vi "PlatMods Artificial.vi"(8 "error in (no error)":errorcluster) -> (0 "error out":errorcluster, 3 "PlatMods":T1)   [LabVIEW 2021, in "RocketPlot.lvlib"]
uses:
  RocketPlot.lvlib
  TypeDefs/PlatMods.ctl
  <vilib>/Utility/inputDevices.llb/keyboardAcquire.vi
  <vilib>/Utility/inputDevices.llb/closeKeyboard.vi
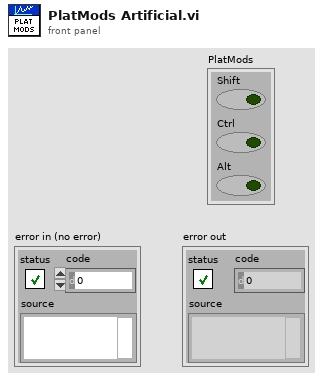
[diagram p1: front panel]
types:
  T1 = typedef "RocketPlot.lvlib/PlatMods.ctl" = cluster{"Shift":bool, "Ctrl":bool, "Alt":bool}
  T2 = enum16{"0", "1", "2", "3", "4", "5", "6", "7", "8", "9", "A", "B", "C", "D", "E", "F", "G", "H", "I", "J", "K", "L", "M", "N", "O", "P", "Q", "R", "S", "T", "U", "V", "W", "X", "Y", "Z", "F1", "F2", "F3", "F4", "F5", "F6", "F7", "F8", "F9", "F10", "F11", "F12", "F13", "F14", "F15", "ADD", "BACK", "BACKSLASH", "CAPITAL", "COMMA", "DECIMAL", "DELETE", "DIVIDE", "DOWN", "END", "EQUALS", "ESCAPE", "GRAVE (`)", "HOME", "INSERT", "LBRACKET", "LCONTROL", "LEFT", "L ALT", "LSHIFT", "LWIN", "MINUS", "MULTIPLY", "NEXT", "NUMLOCK", "NUMPAD_0", "NUMPAD_1", "NUMPAD_2", "NUMPAD_3", "NUMPAD_4", "NUMPAD_5", "NUMPAD_6", "NUMPAD_7", "NUMPAD_8", "NUMPAD_9", "PAUSE", "PERIOD", "PRIOR (PG UP)", "RBRACKET", "RCONTROL", "RETURN", "RIGHT", "R ALT", "RSHIFT", "RWIN", "SCROLL", "SEMICOLON", "SLASH", "SPACE", "SUBTRACT", "TAB", "UP", "ENTER (num pad)", "' (quote)"}
  T3 = enum16{"0", "1", "2", "3", "4", "5", "6", "7", "8", "9", "A", "B", "C", "D", "E", "F", "G", "H", "I", "J", "K", "L", "M", "N", "O", "P", "Q", "R", "S", "T", "U", "V", "W", "X", "Y", "Z", "F1", "F2", "F3", "F4", "F5", "F6", "F7", "F8", "F9", "F10", "F11", "F12", "F13", "F14", "F15", "ADD", "BACK", "BACKSLASH", "CAPITAL", "COMMA", "DECIMAL", "DELETE", "DIVIDE", "DOWN", "END", "EQUALS", "ESCAPE", "GRAVE (`)", "HOME", "INSERT", "LBRACKET", "LCONTROL", "LEFT", "L ALT", "LSHIFT", "LWIN", "MINUS", "MULTIPLY", "NEXT", "NUMLOCK", "NUMPAD_0", "NUMPAD_1", "NUMPAD_2", "NUMPAD_3", "NUMPAD_4", "NUMPAD_5", "NUMPAD_6", "NUMPAD_7", "NUMPAD_8", "NUMPAD_9", "PAUSE", "PERIOD", "PRIOR (PG UP)", "RBRACKET", "RCONTROL", "RETURN", "RIGHT", "R ALT", "RSHIFT", "RWIN", "SCROLL", "SEMICOLON", "SLASH", "SPACE", "SUBTRACT", "TAB", "UP", "ENTER (num pad)", "' (quote)"}[]
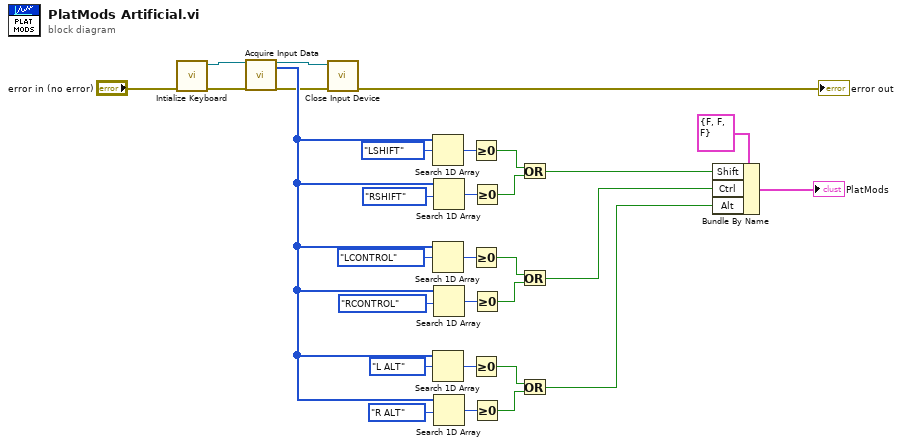
[diagram p0: block diagram]
diagram:
  n1 = call <vilib>:"Intialize Keyboard.vi"("error in (no error)"="error in (no error)") -> ("error out"=w6:errorcluster, "device ID"=w24:refnum<k1>)  [unwired: 9 in]
  n2 = call-poly <vilib>:"Acquire Input Data.vi"("device ID"=w24, "error in (no error)"=w6) -> ("device ID"=w23:refnum<k1>, "keys pressed"=w9:T3, "error out"=w5:errorcluster)  [unwired: 15 in]
  n3 = call-poly <vilib>:"Close Input Device.vi"("error in (no error)"=w5, "device ID"=w23) -> ("error out"=→"error out":errorcluster)  [unwired: 8 in]
  n4 = Search 1D Array(1D array=w9, element=T2."LSHIFT") -> (index of element=w29:i32)  [unwired: 1 in]
  n5 = Search 1D Array(1D array=w9, element=T2."LCONTROL") -> (index of element=w17:i32)  [unwired: 1 in]
  n6 = Search 1D Array(1D array=w9, element=T2."L ALT") -> (index of element=w14:i32)  [unwired: 1 in]
  n7 = Search 1D Array(1D array=w9, element=T2."RSHIFT") -> (index of element=w28:i32)  [unwired: 1 in]
  n8 = Search 1D Array(1D array=w9, element=T2."RCONTROL") -> (index of element=w18:i32)  [unwired: 1 in]
  n9 = Search 1D Array(1D array=w9, element=T2."R ALT") -> (index of element=w13:i32)  [unwired: 1 in]
  n10 = Greater Or Equal To 0?(x=w29) -> (x >= 0?=w27:bool)
  n11 = Greater Or Equal To 0?(x=w17) -> (x >= 0?=w19:bool)
  n12 = Greater Or Equal To 0?(x=w14) -> (x >= 0?=w12:bool)
  n13 = Greater Or Equal To 0?(x=w28) -> (x >= 0?=w26:bool)
  n14 = Greater Or Equal To 0?(x=w18) -> (x >= 0?=w20:bool)
  n15 = Greater Or Equal To 0?(x=w13) -> (x >= 0?=w11:bool)
  n16 = Or(x=w27, y=w26) -> (x .or. y?=w22:bool)
  n17 = Or(x=w19, y=w20) -> (x .or. y?=w8:bool)
  n18 = Or(x=w12, y=w11) -> (x .or. y?=w7:bool)
  n19 = Bundle By Name(cluster=T1 {"Shift"=FALSE, "Ctrl"=FALSE, "Alt"=FALSE} ("PlatMods"), "Shift"=w22, "Ctrl"=w8, "Alt"=w7) -> (→"PlatMods":T1)
